vi "svx_SC Line Data Changed.vi"(4 "probe angles Y":u32=90 max=360 step=1, 6 "probe angles X":u32 max=360 step=1, 9 "DC Y":dbl[](array[numeric]), 11 "DC X":dbl[](array[numeric])) -> (2 "probe angles":cluster{"angles X":dbl, "angles Y":dbl}, 3 "SC Line Data":cluster{"x":dbl[], "y":dbl[]})   [LabVIEW 2017, in "SVX SC Line.xctl"]
uses:
  <vilib>/addons/_XControls/Shaft Centerline/SVX SC Line.xctl
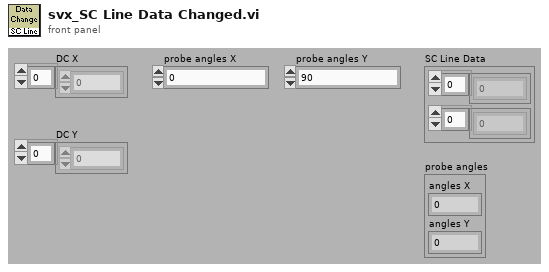
[diagram p1: front panel]
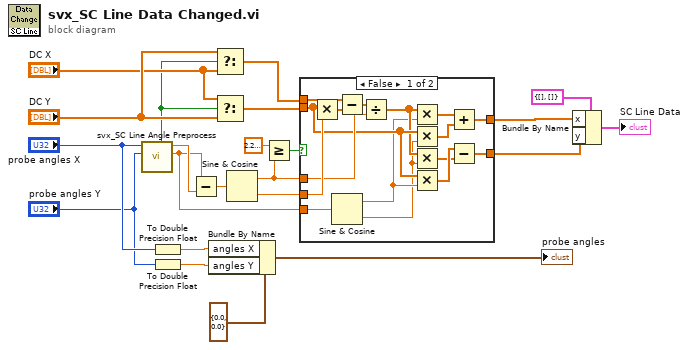
[diagram p0: block diagram]
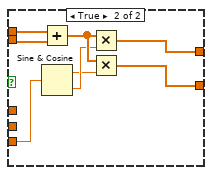
[diagram p2: hidden frame]
diagram:
  n1 = call <vilib>:"svx_SC Line Angle Preprocess.vi"("probe angles Y"="probe angles Y", "probe angles X"="probe angles X") -> ("angles Y"=w8:dbl, "angles X"=w14:dbl, "switch x y axis"=w9:bool)  [unwired: 7 in]
  n2 = To Double Precision Float(number="probe angles X") -> (double precision float=w4:dbl)
  n3 = To Double Precision Float(number="probe angles Y") -> (double precision float=w2:dbl)
  n4 = Subtract(x=w8, y=w14) -> (x-y=w22:dbl)
  n5 = Bundle By Name(cluster=cluster{"angles X":dbl, "angles Y":dbl} {"angles X"=0.0, "angles Y"=0.0} ("probe angles"), "angles X"=w4, "angles Y"=w2) -> (→"probe angles":cluster{"angles X":dbl, "angles Y":dbl})
  n6 = Select(t="DC Y", s=w9, f="DC X") -> (s? t:f=w13:dbl[])
  n7 = Select(t="DC X", s=w9, f="DC Y") -> (s? t:f=w11:dbl[])
  n8 = Sine & Cosine(0:w22) -> (1:w16:dbl, 2:w21:dbl)
  n9 = Greater Or Equal?(x=2.220446049250313e-16, y=w16) -> (x >= y?=w15:bool)
  n10 = case shown="False" w15 {
    tunnel: w21 -> [w38 _]
    tunnel: w16 -> [w36 _]
    tunnel: w8 -> [w31 w43]
    tunnel: w13 -> [w29 w46]
    tunnel: w11 -> [w32 w45]
    tunnel: [w24 w40] -> w20
    tunnel: [w23 w39] -> w19
    frame False {
      n11 = Multiply(x=w32, y=w38) -> (x*y=w35:dbl[])
      n12 = Sine & Cosine(0:w31) -> (1:w26:dbl, 2:w25:dbl)
      n13 = Subtract(x=w29, y=w35) -> (x-y=w37:dbl[])
      n14 = Divide(x=w37, y=w36) -> (x/y=w30:dbl[])
      n15 = Multiply(x=w30, y=w26) -> (x*y=w34:dbl[])
      n16 = Multiply(x=w32, y=w25) -> (x*y=w33:dbl[])
      n17 = Multiply(x=w30, y=w25) -> (x*y=w27:dbl[])
      n18 = Multiply(x=w32, y=w26) -> (x*y=w28:dbl[])
      n19 = Add(x=w34, y=w33) -> (x+y=w24:dbl[])
      n20 = Subtract(x=w28, y=w27) -> (x-y=w23:dbl[])
    }
    frame True {
      n21 = Add(x=w46, y=w45) -> (x+y=w44:dbl[])
      n22 = Sine & Cosine(0:w43) -> (1:w41:dbl, 2:w42:dbl)
      n23 = Multiply(x=w44, y=w42) -> (x*y=w40:dbl[])
      n24 = Multiply(x=w44, y=w41) -> (x*y=w39:dbl[])
    }
  }
  n25 = Bundle By Name(cluster=cluster{"x":dbl[], "y":dbl[]} {"x"=[], "y"=[]} ("output cluster"), "x"=w20, "y"=w19) -> (→"SC Line Data":cluster{"x":dbl[], "y":dbl[]})
